vi "Test FCR100 API.vi"() -> ()   [LabVIEW 2020]
doc: "FCR100 API Tester."
uses:
  Support/Device state -- enum.ctl
  <vilib>/Utility/error.llb/DialogType.ctl
  FCR100.lvlib
panel:
  in  "Interface names":u16(ring) items=["ASRL12  (COM12 - USB-SERIAL CH340)"]
  in  "Resource names":u16(ring) items=["ASRL12::INSTR"]
  in  "Find instruments":bool
  in  "Reset controller":bool
  out "Device state":T1=enum."Configuration"
  out "Position":dbl
  in  "Get current position":bool
  in  "Move relative":bool
  in  "Move absolute":bool
  out "ETA":dbl
  in  "Position":dbl
  in  "Get ETA":bool
  out "Velocity":u16
  in  "Get velocity":bool
  in  "Velocity":u16
  in  "Set velocity":bool
  out "Acceleration":u16
  in  "Get acceleration":bool
  in  "Acceleration":u16
  in  "Set acceleration":bool
  in  "Get state":bool
  in  "Address":u8=1
  in  "Stop movement":bool
  in  "Search Home":bool
  in  "Change disable state":bool
  in  "Enter/(leave)":bool
  in  "Change configuration state":bool
  out "Connected?":bool
  in  "Baud Rate":u32=115200
  in  "Connect with dialog":bool
  in  "Show Diagram on Init":bool
  in  "Run as Singleton?":bool
  in  "Show Block Diagram":bool
  in  "Refresh Modules":bool
  out "Active Modules":string[](array[string])
  in  "Stop Module":bool
  in  "Select Module":i32(ring)=-1 caption="Select Module\nTo send Request to" items=["All"=-1]
  in  "Run New Module":bool
  in  "Hide Module Panel":bool
  in  "Show Module Panel":bool
  out "Status":string
  # "This VI tests the API for the Module."
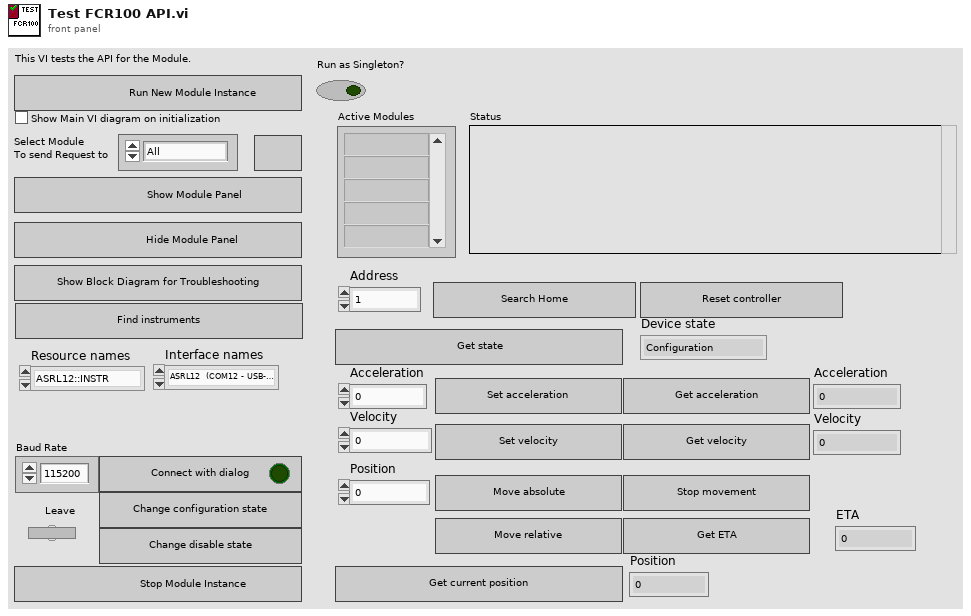
[diagram p1: front panel]
types:
  T1 = typedef "FCR100.lvlib/Device state -- enum.ctl" = enum16{"Not referenced", "Configuration", "Disable", "Ready", "Homing", "Motion"}
  T2 = typedef "FCR100.lvlib/Broadcast Events--cluster.ctl" = cluster{"Module Did Init":refnum<user-event>, "Status Updated":refnum<user-event>, "Error Reported":refnum<user-event>, "Module Did Stop":refnum<user-event>, "Update Module Execution Status":refnum<user-event>, "Device connected":refnum<user-event>, "Connection failed":refnum<user-event>}
  T3 = typedef "DialogType.ctl" = u16
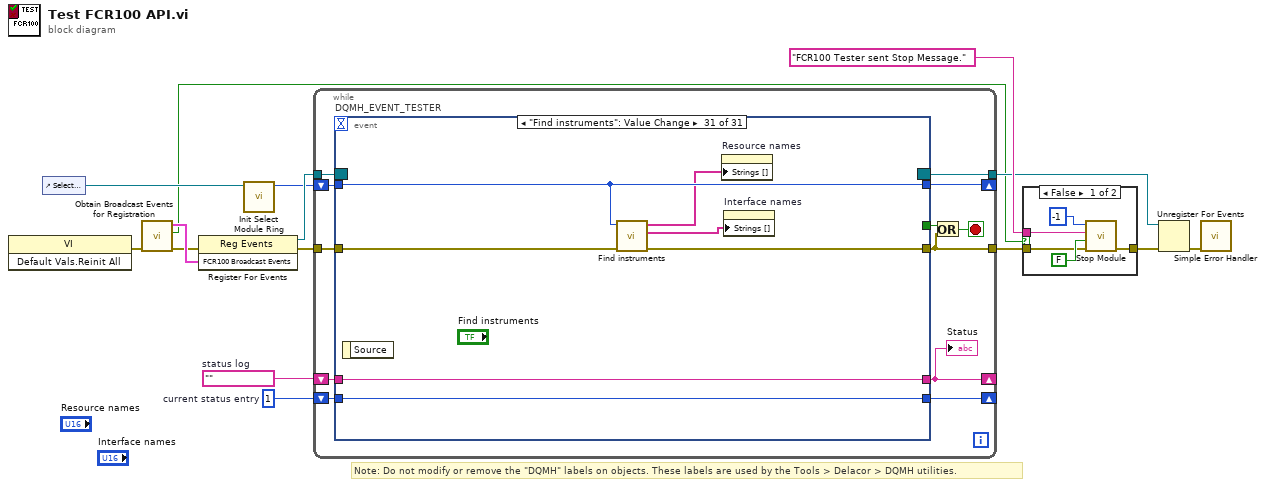
[diagram p0: block diagram]
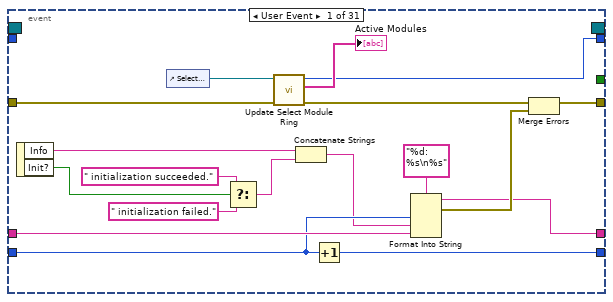
[diagram p3: hidden frame]
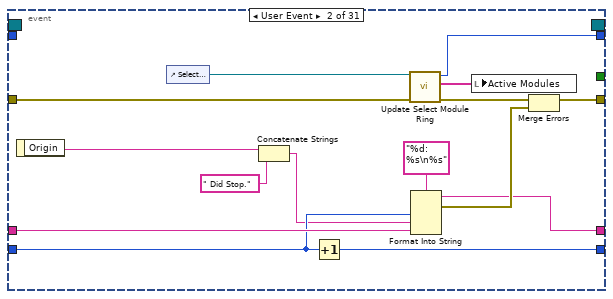
[diagram p4: hidden frame]
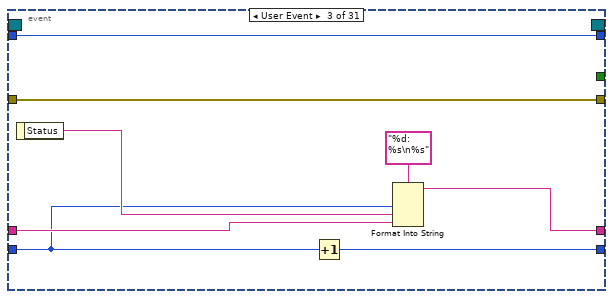
[diagram p5: hidden frame]
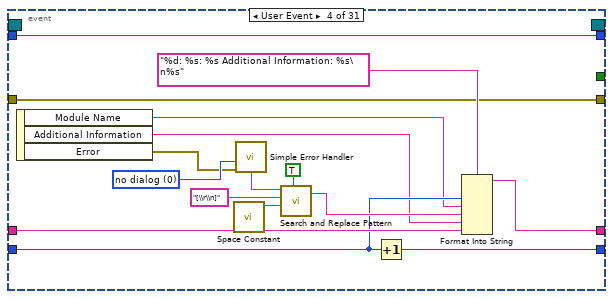
[diagram p6: hidden frame]
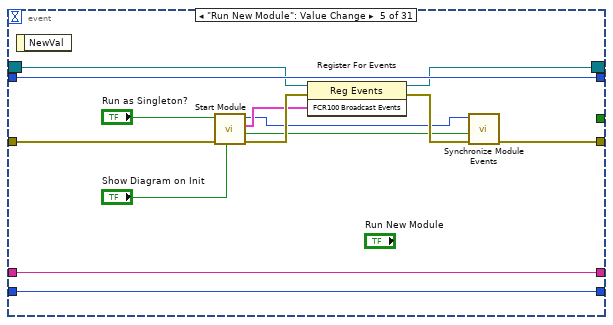
[diagram p7: hidden frame]
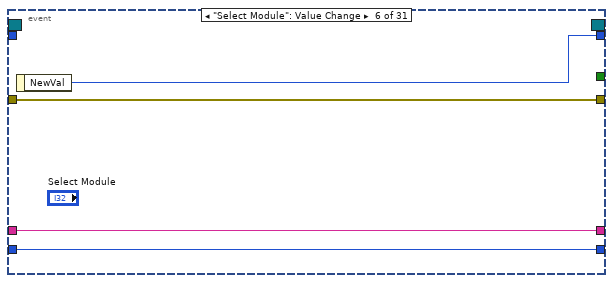
[diagram p8: hidden frame]
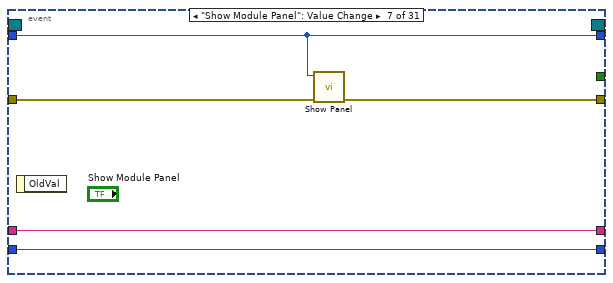
[diagram p9: hidden frame]
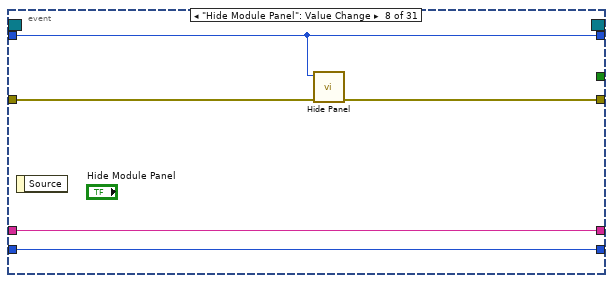
[diagram p10: hidden frame]
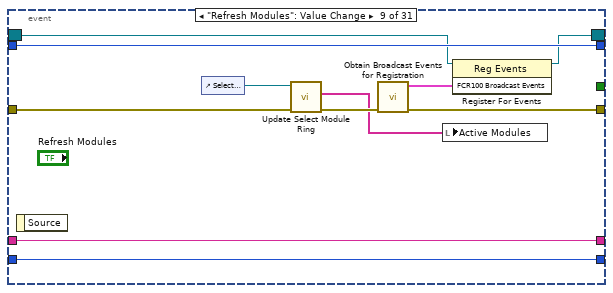
[diagram p11: hidden frame]
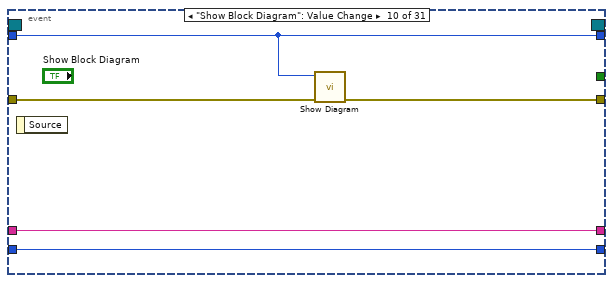
[diagram p12: hidden frame]
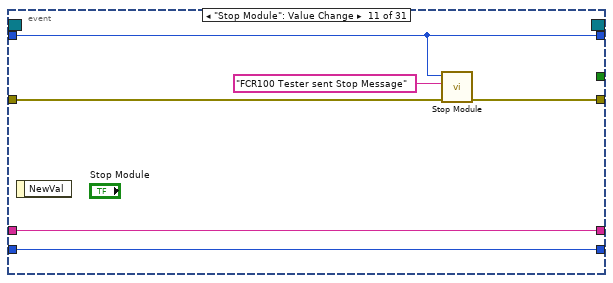
[diagram p13: hidden frame]
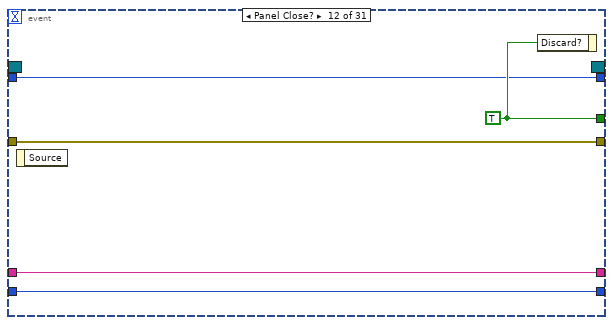
[diagram p14: hidden frame]
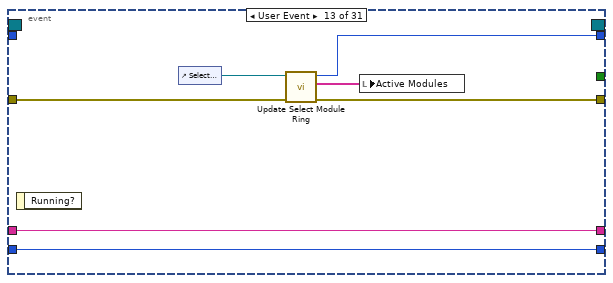
[diagram p15: hidden frame]
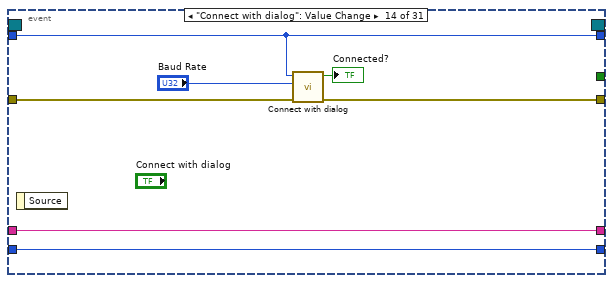
[diagram p16: hidden frame]
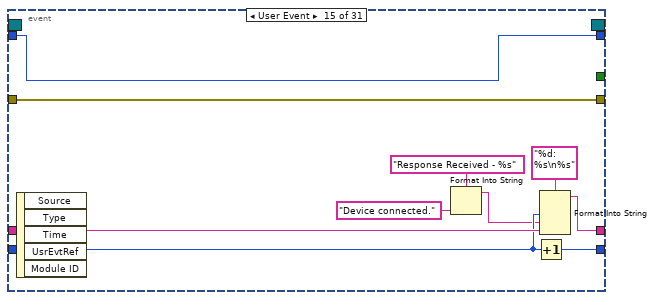
[diagram p17: hidden frame]
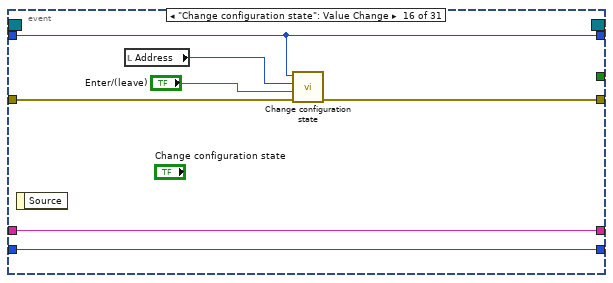
[diagram p18: hidden frame]
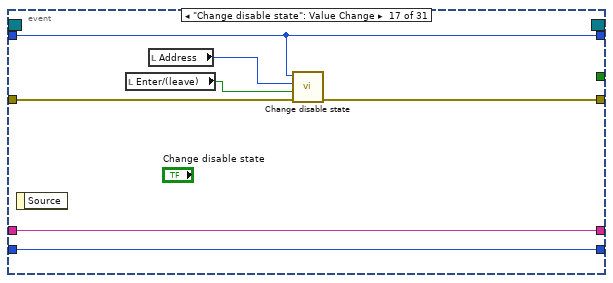
[diagram p19: hidden frame]
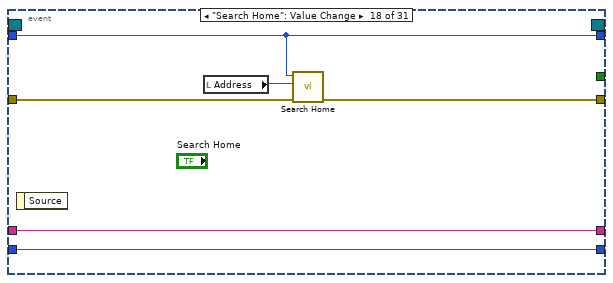
[diagram p20: hidden frame]
diagram:
  w12 = 1  # current status entry
  w13 = ""  # status log
  # "Note: Do not modify or remove the \"DQMH\" labels on objects. These labels are used by the Tools > Delacor > DQMH utilities."
  n1 = invoke class="VI" method="Default Vals.Reinit All"() -> (error out=w5:errorcluster)  [unwired: 3 in, 2 out]
  n2 = control-ref of="Select Module"() -> (w10:refnum<vi>)
  n3 = call "Obtain Broadcast Events for Registration.vi"("error in"=w5) -> ("error out"=w4:errorcluster, "Already running?"=w3:bool, "FCR100 Broadcast Events"=w9:T2)  [unwired: 8 in]
  n4 = register-events(error in=w4, w9) -> (reference out=w15:refnum<event-registration>, error out=w8:errorcluster)  [unwired: 1 in]
  n5 = call "Init Select Module Ring.vi"("Select Module Ring Ref"=w10) -> ("Value for All Modules"=w11:i32)  [unwired: 8 in, 2 out]
  n6 = while {
    tunnel: w15 -> [w27]
    tunnel: [w16] -> w2
    tunnel: w8 -> [w25]
    shift-right: [w21] -> _
    shift-left: w13 -> [w23]
    shift-right: [w22] -> _
    shift-left: w12 -> [w24]
    shift-right: [w18] -> _
    shift-left: w11 -> [w19]
    tunnel: [w17] -> w6
    stop <- w20 stop-if-true
    n7 = event "DQMH_EVENT_TESTER" shown="[30] \"Find instruments\": Value Change" {
      selector: w27 -> [_ _ _ _ w92 _ _ _ w118 _ _ _ _ _ _ _ _ _ _ _ _ _ _ _ _ _ _ _ _ _ _]
      dyn-events: [_ _ _ _ w91 _ _ _ w117 _ _ _ _ _ _ _ _ _ _ _ _ _ _ _ _ _ _ _ _ _ _] -> w17
      timeout: _ -> [_ _ _ _ _ _ _ _ _ _ _ _ _ _ _ _ _ _ _ _ _ _ _ _ _ _ _ _ _ _ _]
      tunnel: [_ _ _ _ _ _ _ _ _ _ _ w139 _ _ _ _ _ _ _ _ _ _ _ _ _ _ _ _ _ _ _] -> w26
      tunnel: [w35 w52 w68 w72 w90 w102 w106 w111 w114 w125 w130 w138 w142 w150 w163 w167 w174 w180 w186 w193 w200 w207 w214 w221 w229 w236 w243 w250 w263 w266 w273] -> w16
      tunnel: w25 -> [w37 w54 w68 w72 w93 w102 w107 w112 w119 w128 w131 w138 w143 w153 w163 w170 w177 w183 w189 w196 w203 w210 w217 w224 w232 w239 w246 w253 w263 w269 w276]
      tunnel: w24 -> [w42 w57 w61 w75 w95 w100 w104 w109 w122 w126 w133 w136 w145 w151 w159 w168 w175 w181 w187 w194 w201 w208 w215 w222 w230 w237 w244 w251 w259 w267 w274]
      tunnel: w23 -> [w43 w58 w64 w76 w96 w101 w105 w110 w123 w127 w134 w137 w146 w152 w161 w169 w176 w182 w188 w195 w202 w209 w216 w223 w231 w238 w245 w252 w261 w268 w275]
      tunnel: [w40 w55 w65 w74 w96 w101 w105 w110 w123 w127 w134 w137 w146 w152 w160 w169 w176 w182 w188 w195 w202 w209 w216 w223 w231 w238 w245 w252 w260 w268 w275] -> w21
      tunnel: [w41 w56 w67 w73 w95 w100 w104 w109 w122 w126 w133 w136 w145 w151 w158 w168 w175 w181 w187 w194 w201 w208 w215 w222 w230 w237 w244 w251 w258 w267 w274] -> w22
      tunnel: w19 -> [_ _ w62 w84 w94 _ w103 w108 w121 w124 w132 w135 _ w149 w162 w166 w173 w179 w185 w192 w199 w206 w213 w220 w227 w235 w242 w248 w262 w265 w272]
      tunnel: [w32 w49 w62 w84 w94 w99 w103 w108 w121 w124 w132 w135 w141 w149 w162 w166 w173 w179 w185 w192 w199 w206 w213 w220 w227 w235 w242 w248 w262 w265 w272] -> w18
      event User Event {
        n8 = event-data() -> ("Info"=w39:string, "Init?"=w29:bool)  [unwired: 1 in]
        n9 = control-ref of="Select Module"() -> (w34:refnum<vi>)
        n10 = Select(t=" initialization succeeded.", s=w29, f=" initialization failed.") -> (s? t:f=w28:string)
        n11 = call "Update Select Module Ring.vi"("error in (no error)"=w37, "Select Module Ring Ref"=w34) -> ("error out"=w36:errorcluster, "Active Modules (Array)"=→"Active Modules":string[], "New Module Ring Value"=w32:i32)  [unwired: 7 in]
        n12 = Concatenate Strings(w39, w28) -> (w38:string)
        n13 = Increment(x=w42) -> (x+1=w41:i32)
        n14 = Format Into String(format string="%d: %s\n%s", w42, w38, w43) -> (resulting string=w40:string, error out=w45:errorcluster)  [unwired: 2 in]
        n15 = Merge Errors(w36, w45) -> (w35:errorcluster)
      }
      event User Event {
        n16 = event-data() -> ("Origin"=w47:string)  [unwired: 1 in]
        n17 = control-ref of="Select Module"() -> (w51:refnum<vi>)
        n18 = Concatenate Strings(w47, " Did Stop.") -> (w46:string)
        n19 = Increment(x=w57) -> (x+1=w56:i32)
        n20 = call "Update Select Module Ring.vi"("error in (no error)"=w54, "Select Module Ring Ref"=w51) -> ("error out"=w53:errorcluster, "Active Modules (Array)"=w50:string[], "New Module Ring Value"=w49:i32)  [unwired: 7 in]
        n21 = Format Into String(format string="%d: %s\n%s", w57, w46, w58) -> (resulting string=w55:string, error out=w60:errorcluster)  [unwired: 2 in]
        n22 = local write "Active Modules"(w50) -> ()
        n23 = Merge Errors(w53, w60) -> (w52:errorcluster)
      }
      event User Event {
        n24 = event-data() -> ("Status"=w63:string)  [unwired: 1 in]
        n25 = Increment(x=w61) -> (x+1=w67:i32)
        n26 = Format Into String(format string="%d: %s\n%s", w61, w63, w64) -> (resulting string=w65:string)  [unwired: 2 in, 1 out]
      }
      event User Event {
        w77 = T3 0 items=["no dialog", "OK message", "continue or stop message", "OK message + warnings", "continue/stop + warnings"] ("type of dialog (OK msg:1)")
        n27 = event-data() -> ("Module Name"=w71:string, "Additional Information"=w70:string, "Error"=w69:errorcluster)  [unwired: 1 in]
        n28 = call <vilib>:"Space Constant.vi"() -> ("String"=w81:string)
        n29 = call <vilib>:"Simple Error Handler.vi"("type of dialog (OK msg:1)"=w77, "error in (no error)"=w69) -> ("message"=w78:string)  [unwired: 3 in, 4 out]
        n30 = call <vilib>:"Search and Replace Pattern.vi"("string"=w78, "regular expression (\"\")"="[\\r\\n]" ("regular expression (\"\")"), "replace string (\"\")"=w81, "replace all? (F)"=TRUE ("replace all CR/LF with spaces")) -> ("result string"=w79:string)  [unwired: 1 in, 1 out]
        n31 = Increment(x=w75) -> (x+1=w73:i32)
        n32 = Format Into String(format string="%d: %s: %s Additional Information: %s\n%s", w75, w71, w79, w70, w76) -> (resulting string=w74:string)  [unwired: 2 in, 1 out]
      }
      event "Run New Module": Value Change {
        n33 = event-data() -> ()  [unwired: 1 in, 1 out]
        n34 = call "Start Module.vi"("Show Main VI Diagram on Init (F)"="Show Diagram on Init", "error in"=w93, "Run as Singleton? (F)"="Run as Singleton?") -> ("error out"=w97:errorcluster, "Wait for Event Sync?"=w89:bool, "FCR100 Broadcast Events"=w88:T2, "Module ID"=w85:i32)  [unwired: 5 in]
        n35 = register-events(reference=w92, error in=w97, w88) -> (reference out=w91:refnum<event-registration>, error out=w98:errorcluster)
        n36 = call "Synchronize Module Events.vi"("error in"=w98, "Wait for Event Sync?"=w89, "Module ID in"=w85) -> ("error out"=w90:errorcluster)  [unwired: 7 in, 1 out]
      }
      event "Select Module": Value Change {
        n37 = event-data() -> ("NewVal"=w99:i32)  [unwired: 1 in]
      }
      event "Show Module Panel": Value Change {
        n38 = event-data() -> ()  [unwired: 1 in, 1 out]
        n39 = call "Show Panel.vi"("error in (no error)"=w107, "Module ID"=w103) -> ("error out"=w106:errorcluster)  [unwired: 9 in]
      }
      event "Hide Module Panel": Value Change {
        n40 = event-data() -> ()  [unwired: 1 in, 1 out]
        n41 = call "Hide Panel.vi"("error in (no error)"=w112, "Module ID"=w108) -> ("error out"=w111:errorcluster)  [unwired: 9 in]
      }
      event "Refresh Modules": Value Change {
        n42 = event-data() -> ()  [unwired: 1 in, 1 out]
        n43 = control-ref of="Select Module"() -> (w120:refnum<vi>)
        n44 = call "Update Select Module Ring.vi"("error in (no error)"=w119, "Select Module Ring Ref"=w120) -> ("error out"=w115:errorcluster, "Active Modules (Array)"=w113:string[])  [unwired: 7 in, 1 out]
        n45 = call "Obtain Broadcast Events for Registration.vi"("error in"=w115) -> ("error out"=w114:errorcluster, "FCR100 Broadcast Events"=w116:T2)  [unwired: 8 in, 1 out]
        n46 = local write "Active Modules"(w113) -> ()
        n47 = register-events(reference=w118, w116) -> (reference out=w117:refnum<event-registration>)  [unwired: 1 in, 1 out]
      }
      event "Show Block Diagram": Value Change {
        n48 = event-data() -> ()  [unwired: 1 in, 1 out]
        n49 = call "Show Diagram.vi"("error in (no error)"=w128, "Module ID"=w124) -> ("error out"=w125:errorcluster)  [unwired: 9 in]
      }
      event "Stop Module": Value Change {
        n50 = event-data() -> ()  [unwired: 1 in, 1 out]
        n51 = call "Stop Module.vi"("error in"=w131, "Origin"="FCR100 Tester sent Stop Message", "Module ID"=w132) -> ("error out"=w130:errorcluster)  [unwired: 8 in]
      }
      event Panel Close? {
        w139 = TRUE ("Discard?")
        n52 = event-data() -> ()  [unwired: 1 in, 1 out]
        n53 = event-data("Discard?"=w139) -> ()  [unwired: 1 in, 1 out]
      }
      event User Event {
        n54 = event-data() -> ()  [unwired: 1 in, 1 out]
        n55 = control-ref of="Select Module"() -> (w144:refnum<vi>)
        n56 = call "Update Select Module Ring.vi"("error in (no error)"=w143, "Select Module Ring Ref"=w144) -> ("error out"=w142:errorcluster, "Active Modules (Array)"=w140:string[], "New Module Ring Value"=w141:i32)  [unwired: 7 in]
        n57 = local write "Active Modules"(w140) -> ()
      }
      event "Connect with dialog": Value Change {
        n58 = event-data() -> ()  [unwired: 1 in, 1 out]
        n59 = call "Connect with dialog.vi"("error in"=w153, "Baud Rate (115200 - USB)"="Baud Rate", "Module ID"=w149) -> ("error out"=w150:errorcluster, "Connected?"=→"Connected?":bool)  [unwired: 6 in, 1 out]
      }
      event User Event {
        n60 = event-data() -> ()  [unwired: 1 in, 5 out]
        n61 = Format Into String(format string="Response Received - %s", "Device connected." ("input 1")) -> (resulting string=w155:string)  [unwired: 2 in, 1 out]
        n62 = Increment(x=w159) -> (x+1=w158:i32)
        n63 = Format Into String(format string="%d: %s\n%s", w159, w155, w161) -> (resulting string=w160:string)  [unwired: 2 in, 1 out]
      }
      event "Change configuration state": Value Change {
        n64 = event-data() -> ()  [unwired: 1 in, 1 out]
        n65 = local read "Address"() -> (w164:u8)
        n66 = call "Change configuration state.vi"("error in"=w170, "Enter/(leave)"="Enter/(leave)", "Address"=w164, "Module ID"=w166) -> ("error out"=w167:errorcluster)  [unwired: 7 in]
      }
      event "Change disable state": Value Change {
        n67 = event-data() -> ()  [unwired: 1 in, 1 out]
        n68 = local read "Enter/(leave)"() -> (w172:bool)
        n69 = local read "Address"() -> (w171:u8)
        n70 = call "Change disable state.vi"("error in"=w177, "Enter/Leave"=w172, "Address"=w171, "Module ID"=w173) -> ("error out"=w174:errorcluster)  [unwired: 7 in]
      }
      event "Search Home": Value Change {
        n71 = event-data() -> ()  [unwired: 1 in, 1 out]
        n72 = local read "Address"() -> (w178:u8)
        n73 = call "Search Home.vi"("error in"=w183, "Address"=w178, "Module ID"=w179) -> ("error out"=w180:errorcluster)  [unwired: 8 in]
      }
      event "Stop movement": Value Change {
        n74 = event-data() -> ()  [unwired: 1 in, 1 out]
        n75 = call "Stop movement.vi"("error in"=w189, "Address"="Address", "Module ID"=w185) -> ("error out"=w186:errorcluster)  [unwired: 8 in]
      }
      event "Get state": Value Change {
        n76 = event-data() -> ()  [unwired: 1 in, 1 out]
        n77 = local read "Address"() -> (w191:u8)
        n78 = call "Get state.vi"("error in"=w196, "Address"=w191, "Module ID"=w192) -> ("error out"=w193:errorcluster, "Device state"=→"Device state":T1)  [unwired: 6 in, 1 out]
      }
      event "Set acceleration": Value Change {
        n79 = event-data() -> ()  [unwired: 1 in, 1 out]
        n80 = local read "Address"() -> (w198:u8)
        n81 = call "Set acceleration.vi"("error in"=w203, "Acceleration"="Acceleration", "Address"=w198, "Module ID"=w199) -> ("error out"=w200:errorcluster)  [unwired: 7 in]
      }
      event "Get acceleration": Value Change {
        n82 = event-data() -> ()  [unwired: 1 in, 1 out]
        n83 = local read "Address"() -> (w205:u8)
        n84 = call "Get acceleration.vi"("error in"=w210, "Address"=w205, "Module ID"=w206) -> ("error out"=w207:errorcluster, "Acceleration"=→"Acceleration":u16)  [unwired: 6 in, 1 out]
      }
      event "Set velocity": Value Change {
        n85 = event-data() -> ()  [unwired: 1 in, 1 out]
        n86 = local read "Address"() -> (w212:u8)
        n87 = call "Set velocity.vi"("error in"=w217, "Velocity"="Velocity", "Address"=w212, "Module ID"=w213) -> ("error out"=w214:errorcluster)  [unwired: 7 in]
      }
      event "Get velocity": Value Change {
        n88 = event-data() -> ()  [unwired: 1 in, 1 out]
        n89 = local read "Address"() -> (w219:u8)
        n90 = call "Get velocity.vi"("error in"=w224, "Address"=w219, "Module ID"=w220) -> ("error out"=w221:errorcluster, "Velocity"=→"Velocity":u16)  [unwired: 6 in, 1 out]
      }
      event "Get ETA": Value Change {
        n91 = event-data() -> ()  [unwired: 1 in, 1 out]
        n92 = local read "Address"() -> (w228:u8)
        n93 = call "Get ETA.vi"("error in"=w232, "Position"="Position", "Address"=w228, "Module ID"=w227) -> ("error out"=w229:errorcluster, "ETA"=→"ETA":dbl)  [unwired: 5 in, 1 out]
      }
      event "Move absolute": Value Change {
        n94 = event-data() -> ()  [unwired: 1 in, 1 out]
        n95 = local read "Address"() -> (w234:u8)
        n96 = local read "Position"() -> (w233:dbl)
        n97 = call "Move absolute.vi"("error in"=w239, "Position"=w233, "Numeric"=w234, "Module ID"=w235) -> ("error out"=w236:errorcluster)  [unwired: 7 in]
      }
      event "Move relative": Value Change {
        n98 = event-data() -> ()  [unwired: 1 in, 1 out]
        n99 = local read "Address"() -> (w241:u8)
        n100 = local read "Position"() -> (w240:dbl)
        n101 = call "Move relative.vi"("error in"=w246, "Position"=w240, "Address"=w241, "Module ID"=w242) -> ("error out"=w243:errorcluster)  [unwired: 7 in]
      }
      event "Get current position": Value Change {
        n102 = event-data() -> ()  [unwired: 1 in, 1 out]
        n103 = local read "Address"() -> (w249:u8)
        n104 = call "Get current position.vi"("error in"=w253, "Address"=w249, "Module ID"=w248) -> ("error out"=w250:errorcluster, "Position"=→"Position":dbl)  [unwired: 6 in, 1 out]
      }
      event User Event {
        n105 = event-data() -> ()  [unwired: 1 in, 5 out]
        n106 = Format Into String(format string="Response Received - %s", "Connection failed." ("input 1")) -> (resulting string=w255:string)  [unwired: 2 in, 1 out]
        n107 = Increment(x=w259) -> (x+1=w258:i32)
        n108 = Format Into String(format string="%d: %s\n%s", w259, w255, w261) -> (resulting string=w260:string)  [unwired: 2 in, 1 out]
      }
      event "Reset controller": Value Change {
        n109 = event-data() -> ()  [unwired: 1 in, 1 out]
        n110 = local read "Address"() -> (w264:u8)
        n111 = call "Reset controller.vi"("error in"=w269, "Address"=w264, "Module ID"=w265) -> ("error out"=w266:errorcluster)  [unwired: 8 in]
      }
      event "Find instruments": Value Change {
        n112 = event-data() -> ()  [unwired: 1 in, 1 out]
        n113 = call "Find instruments.vi"("error in"=w276, "Module ID"=w272) -> ("error out"=w273:errorcluster, "Interface Names"=w270:string[], "Resource Names"=w271:string[])  [unwired: 6 in, 1 out]
        n114 = property on="Resource names" class="Ring (strict)"("Strings []"=w271) -> ()  [unwired: 2 in, 2 out]
        n115 = property on="Interface names" class="Ring (strict)"("Strings []"=w270) -> ()  [unwired: 2 in, 2 out]
      }
    }
    "Status" <- w21
    n116 = Or(x=w26, y=w16) -> (x .or. y?=w20:bool)
  }
  n117 = case shown="False" w3 {
    tunnel: [w281 w282] -> w14
    tunnel: "FCR100 Tester sent Stop Message." ("Origin") -> [w280 _]
    tunnel: w2 -> [w277 w282]
    frame False {
      n118 = call "Stop Module.vi"("error in"=w277, "Wait for Module to stop? (F)"=FALSE ("Wait for Module to stop?"), "Origin"=w280, "Module ID"=-1 ("Stop all")) -> ("error out"=w281:errorcluster)  [unwired: 7 in]
    }
    frame True {
    }
  }
  n119 = Unregister For Events(event registration refnum=w6, error in=w14) -> (error out=w1:errorcluster)
  n120 = call <vilib>:"Simple Error Handler.vi"("error in (no error)"=w1) -> ()  [unwired: 4 in, 5 out]
